vi "clear map.vi"   [LabVIEW 2015]
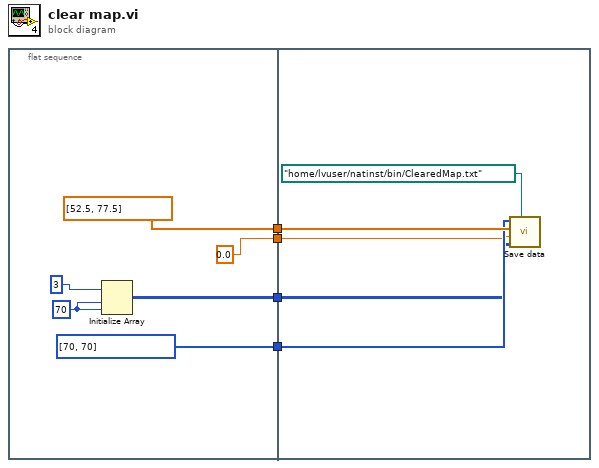
[diagram p0: block diagram]
diagram:
  n1 = flat-sequence {
    tunnel: [dbl[] [52.5, 77.5]] -> w4
    tunnel: [i32[] [70, 70]] -> w3
    tunnel: [w6] -> w2
    tunnel: [0.0] -> w1
    tunnel: w4 -> [w14]
    tunnel: w3 -> [w13]
    tunnel: w2 -> [w12]
    tunnel: w1 -> [w11]
    frame #0 {
      w8 = 70
      n2 = Initialize Array(3, w8, w8) -> (w6:i32[][])
    }
    frame #1 {
      n3 = call "Save data.vi"("file path (use dialog)"=path "/home/lvuser/natinst/bin/ClearedMap.txt", "Obsticle map"=w12, "Robot angle"=w11, "Actual robot location"=w14, "Map dimensions"=w13) -> ()  [unwired: 7 in]
    }
  }
